vi "VS Compute Waveform.vi"(0 "number of points (1000)":i32=1000, 1 "signal type (0:sine)":T1(ring) caption="signal type (0:dc)", 5 "amplitude (1.0)":dbl=1.0 format="%.2f", 7 "offset (0.0)":dbl format="%.2f", 9 "phase (0 deg)":dbl format="%.2f", 11 "error in (no error)":errorcluster, 12 "% duty cycle\n(square wave only, 50)":i32=50) -> (6 "waveform graph":dbl[](graph), 15 "error out":errorcluster)   [LabVIEW 2013]
doc: "This is a subVI used by the function generator analog output example.\n\nThis VI computes a single cycle of a waveform - square, sine, triangle or sawtooth with the number of points, amplitude, offset and phase specified. The single output waveform is put into a transposed 2D array so that it can be fed directly into the AO Write VI.\n\nNote: for multiple channel waveform generation, the output should be modified as a 1D array so that multiple waveforms can be strung together with an array builder VI."
panel:
  # "Copyright © 2003, Viewpoint Systems Inc.\nAll Rights Reserved\nwww.viewpointusa.com\n(585)-475-9555\nAuthor: Stuart R. McFarlane"
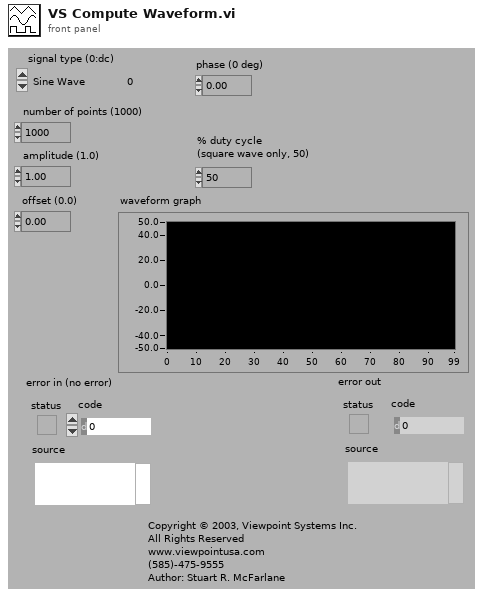
[diagram p1: front panel]
types:
  T1 = enum16{"Sine Wave", "Square Wave", "Sawtooth", "Triangle Wave"}
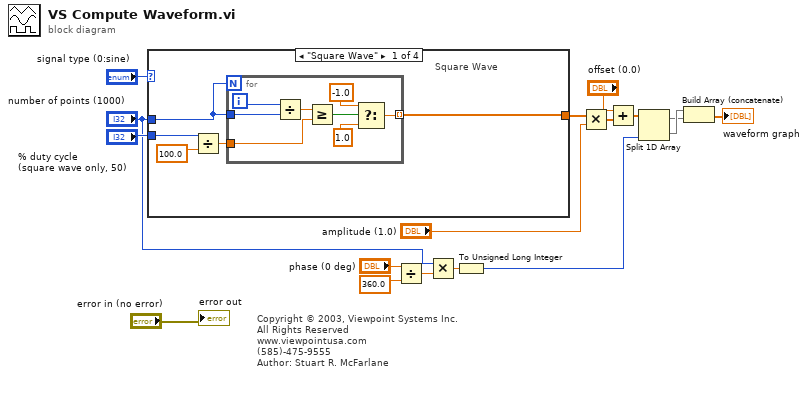
[diagram p0: block diagram]
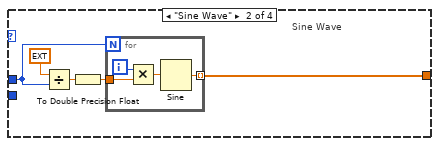
[diagram p2: hidden frame]
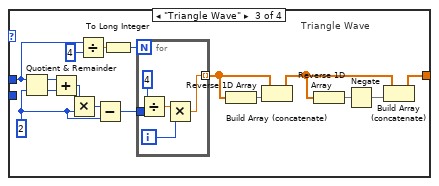
[diagram p3: hidden frame]
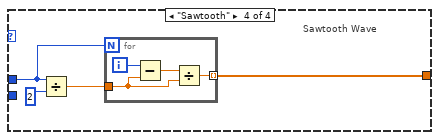
[diagram p4: hidden frame]
diagram:
  # "Copyright © 2003, Viewpoint Systems Inc.\nAll Rights Reserved\nwww.viewpointusa.com\n(585)-475-9555\nAuthor: Stuart R. McFarlane"
  n1 = case shown="\"Square Wave\"" "signal type (0:sine)" {
    tunnel: "number of points (1000)" -> [w22 w33 w49 w64]
    tunnel: [w18 w32 w44 w61] -> w15
    tunnel: "% duty cycle\n(square wave only, 50)" -> [w21 _ _ _]
    frame "Square Wave" {
      # "Square Wave"
      n2 = Divide(x=w21, y=100.0) -> (x/y=w19:dbl)
      n3 = for {
        N: w22 -> [_]
        tunnel: w22 -> [w29]
        tunnel: w19 -> [w24]
        tunnel: [w23] -> w18 mode=indexing
        i -> [w30]
        n4 = Divide(x=w30, y=w29) -> (x/y=w28:dbl)
        n5 = Greater Or Equal?(x=w28, y=w24) -> (x >= y?=w25:bool)
        n6 = Select(t=-1.0, s=w25, f=1.0) -> (s? t:f=w23:dbl)
      }
    }
    frame "Sine Wave" {
      # "Sine Wave"
      n7 = Divide(x=ext 6.283185307179586477, y=w33) -> (x/y=w34:ext)
      n8 = To Double Precision Float(number=w34) -> (double precision float=w31:dbl)
      n9 = for {
        N: w33 -> [_]
        tunnel: w31 -> [w37]
        tunnel: [w36] -> w32 mode=indexing
        i -> [w38]
        n10 = Multiply(x=w38, y=w37) -> (x*y=w39:dbl)
        n11 = Sine(x=w39) -> (sin(x)=w36:dbl)
      }
    }
    frame "Triangle Wave" {
      w53 = 2
      # "Triangle Wave"
      n12 = Quotient & Remainder(x=w49, y=w53) -> (x-y*floor(x/y)=w52:i32, floor(x/y)=w55:i32)
      n13 = Add(x=w52, y=w55) -> (x+y=w50:i32)
      n14 = Multiply(x=w50, y=w53) -> (x*y=w54:i32)
      n15 = Divide(x=w49, y=4) -> (x/y=w47:dbl)
      n16 = Subtract(x=w54, y=w53) -> (x-y=w51:i32)
      n17 = To Long Integer(number=w47) -> (32bit integer=w46:i32)
      n18 = for {
        N: w46 -> [_]
        tunnel: [w56] -> w41 mode=indexing
        tunnel: w51 -> [w60]
        i -> [w58]
        n19 = Divide(x=4, y=w60) -> (x/y=w57:dbl)
        n20 = Multiply(x=w57, y=w58) -> (x*y=w56:dbl)
      }
      n21 = Reverse 1D Array(array=w41) -> (reversed array=w40:dbl[])
      n22 = Build Array (concatenate)(w41, w40) -> (w43:dbl[])
      n23 = Reverse 1D Array(array=w43) -> (reversed array=w45:dbl[])
      n24 = Negate(x=w45) -> (-x=w42:dbl[])
      n25 = Build Array (concatenate)(w43, w42) -> (w44:dbl[])
    }
    frame "Sawtooth" {
      # "Sawtooth Wave"
      n26 = Divide(x=w64, y=2) -> (x/y=w62:dbl)
      n27 = for {
        N: w64 -> [_]
        tunnel: [w68] -> w61 mode=indexing
        tunnel: w62 -> [w65]
        i -> [w66]
        n28 = Subtract(x=w66, y=w65) -> (x-y=w67:dbl)
        n29 = Divide(x=w67, y=w65) -> (x/y=w68:dbl)
      }
    }
  }
  n30 = Divide(x="phase (0 deg)", y=360.0) -> (x/y=w9:dbl)
  n31 = Multiply(x="number of points (1000)", y=w9) -> (x*y=w7:dbl)
  n32 = To Unsigned Long Integer(number=w7) -> (unsigned 32bit integer=w6:u32)
  n33 = Multiply(x=w15, y="amplitude (1.0)") -> (x*y=w13:dbl[])
  n34 = Add(x="offset (0.0)", y=w13) -> (x+y=w4:dbl[])
  n35 = Split 1D Array(array=w4, index=w6) -> (first subarray=w2:dbl[], second subarray=w3:dbl[])
  n36 = Build Array (concatenate)(w3, w2) -> (→"waveform graph":dbl[])
  "error out" <- "error in (no error)"
